vi "Get Automatic Gain Mode.vi"(8 "error in (no error)":errorcluster, 11 "Stream":refnum<data-value>) -> (0 "error out":errorcluster, 1 "Is Supported":bool, 2 "Automatic Parameter Mode":T1, 3 "Stream (duplicate)":refnum<data-value>)   [LabVIEW 2020, in "g_ar_toolkit.capture.lvlib" / "CameraStream.lvclass"]
uses:
  CameraStream.lvclass
  Camera Automatic Parameter Mode.ctl
  Camera Automatic Parameters.ctl
  CameraStream.lvclass/CameraStream.ctl
  <vilib>/Utility/error.llb/Error Cluster From Error Code.vi
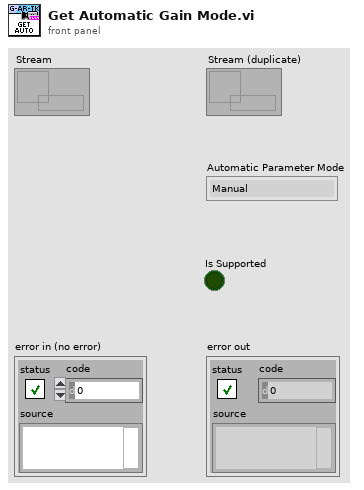
[diagram p1: front panel]
types:
  T1 = typedef "g_ar_toolkit.capture.lvlib/CameraStream.lvclass/Camera Automatic Parameter Mode.ctl" = enum16{"Manual", "Automatic"}
  T2 = typedef "g_ar_toolkit.capture.lvlib/CameraStream.lvclass/Camera Automatic Parameters.ctl" = enum16{"AUTO_EXPOSURE", "AUTO_FOCUS", "AUTO_WHITEBALANCE", "AUTO_GAIN"}
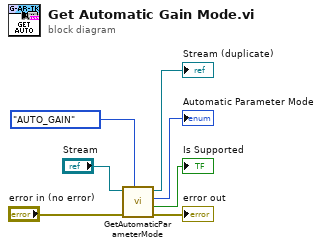
[diagram p0: block diagram]
diagram:
  n1 = call "GetAutomaticParameterMode.vi"("Auto Parameter"=Camera_Automatic_Parameters."AUTO_GAIN", "error in (no error)"="error in (no error)", "Stream"="Stream") -> ("error out"=→"error out":errorcluster, "Is Supported"=→"Is Supported":bool, "Automatic Parameter Mode"=→"Automatic Parameter Mode":T1, "Stream (duplicate)"=→"Stream (duplicate)":refnum<data-value>)  [unwired: 5 in]
